vi "Reset.vi"   [LabVIEW 2013]
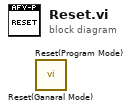
[diagram p0: block diagram]
diagram:
  n1 = call "Reset(Ganaral Mode).vi"() -> ()  [unwired: 10 in, 2 out]
  n2 = call "Reset(Program Mode).vi"() -> ()  [unwired: 10 in, 2 out]
